vi "SWITCH Disconnect.vi"(8 "error in (no error)":errorcluster, 11 "Hardware Resources in":T1={"Tango HW"={"VISA resource"="", "Baud Rate (115200)"=2, "lAnInterfaceType"=0, "bAShowProt"=15}, "Writer Queue"=refnum, "Status"=FALSE, "Abs Position"=[], "Axis Velocity"={"dX"=0.0, "dY"=0.0, "dZ"=0.0, "dA"=0.0}, "acceleration "=0.0, "Z direction"=enum."Up", "Position Mode"="", "plLSID"=0}) -> (0 "error out":errorcluster)   [LabVIEW 2020, in "MOTOR.lvlib"]
doc: "Stops the acquisition."
uses:
  MOTOR.lvlib
  PS Hardware Configuration.ctl
  support/Message Queue/Message Cluster.ctl
  <instrlib>/Tango_DLL/Tango_DLL.lvlib
  support/Message Queue/Message Queue.lvlib
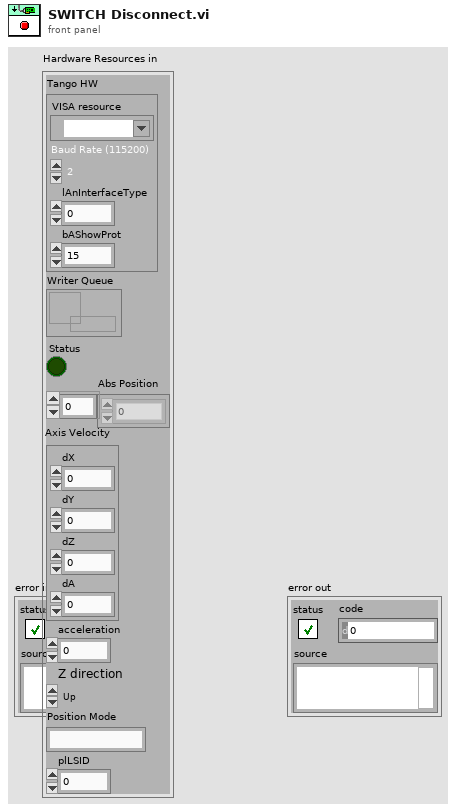
[diagram p1: front panel]
types:
  T1 = typedef "MOTOR.lvlib/PS Hardware Configuration.ctl" = cluster{"Tango HW":cluster{"VISA resource":refnum<visa-resource-name>, "Baud Rate (115200)":i32, "lAnInterfaceType":i32, "bAShowProt":i32}, "Writer Queue":refnum<queue>, "Status":bool, "Abs Position":i32[], "Axis Velocity":cluster{"dX":dbl, "dY":dbl, "dZ":dbl, "dA":dbl}, "acceleration ":dbl, "Z direction":enum16{"Up", "Down"}, "Position Mode":string, "plLSID":i32}
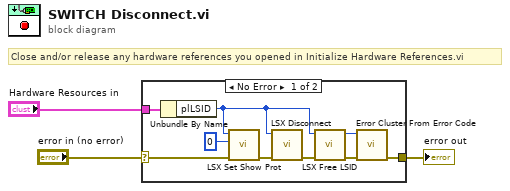
[diagram p0: block diagram]
diagram:
  # "Close and/or release any hardware references you opened in Initialize Hardware References.vi"
  n1 = case shown="No Error" "error in (no error)" {
    selector: "error in (no error)" -> [w6 w13]
    tunnel: [w12 w13] -> w2
    tunnel: "Hardware Resources in" -> [w8 _]
    frame No Error {
      n2 = Unbundle By Name(w8) -> ("plLSID"=w7:i32)
      n3 = call <instrlib>:"LSX Set Show Prot.vi"("error in (no error)"=w6, "bShowProt"=0, "lLSID"=w7) -> ("error out"=w10:errorcluster)  [unwired: 7 in, 1 out]
      n4 = call <instrlib>:"LSX Disconnect.vi"("error in (no error)"=w10, "lLSID"=w7) -> ("error out"=w9:errorcluster)  [unwired: 8 in, 1 out]
      n5 = call <instrlib>:"LSX Free LSID.vi"("error in (no error)"=w9, "lLSID"=w7) -> ("error out"=w5:errorcluster, "function return"=w4:i32)  [unwired: 8 in]
      n6 = call <vilib>:"Error Cluster From Error Code.vi"("error in (no error)"=w5, "error code (0)"=w4) -> ("error out"=w12:errorcluster)  [unwired: 7 in]
    }
    frame Error {
    }
  }
  "error out" <- w2
